vi "Write Trigger Detection.vi"(9 "Write DRAM enable?":bool, 10 "Start address(line) in":u32, 11 "Start address(frame) in":u32) -> (2 "Start address(line) out":u32, 3 "Next Status":enum16{"Wait on Trigger", "Write DRAM"}(ring))   [LabVIEW 2015]
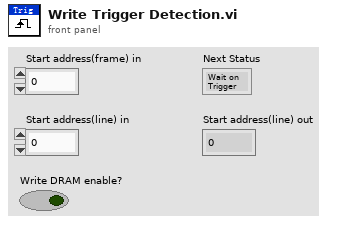
[diagram p1: front panel]
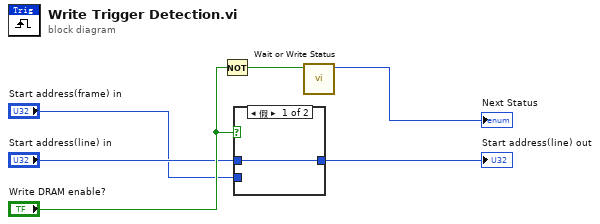
[diagram p0: block diagram]
diagram:
  n1 = Not(x="Write DRAM enable?") -> (.not. x?=w5:bool)
  n2 = case shown="假" "Write DRAM enable?" {
    tunnel: "Start address(frame) in" -> [_ w8]
    tunnel: "Start address(line) in" -> [w7 _]
    tunnel: [w7 w8] -> w3
    frame False {
    }
    frame True {
    }
  }
  "Start address(line) out" <- w3
  n3 = call "Wait or Write Status.vi"("bool in"=w5) -> ("Next Status"=→"Next Status":enum16{"Wait on Trigger", "Write DRAM"})  [unwired: 10 in]
